vi "Pin Query Context to Channel List.vi"(0 "Pin Query Context":refnum<class "PinQueryContext.lvclass">, 5 "Expanded Pin Information":T1[](array[typedef]), 9 "Site Numbers In":i32[](array[numeric]), 11 "error in":errorcluster) -> (4 "Per-Session Channel List":string[](array[string]), 6 "Pins":tag[](array[tag]), 10 "Site Numbers Out":i32[](array[numeric]), 15 "error out":errorcluster)   [LabVIEW 2020]
uses:
  <vilib>/NI_TestStand_SemiconductorModule/NI_TestStand_Semiconductor_Module.lvlibp/PinMap/PinQueryContext/PinQueryContext.lvclass
  TSM Expanded Pin Information.ctl
  TSM Pin Type Identifier.ctl
  <vilib>/NI_TestStand_SemiconductorModule/NI_TestStand_Semiconductor_Module.lvlibp/PinMap/Advanced/GetPinsInPinGroups.vi
  <vilib>/NI_TestStand_SemiconductorModule/NI_TestStand_Semiconductor_Module.lvlibp
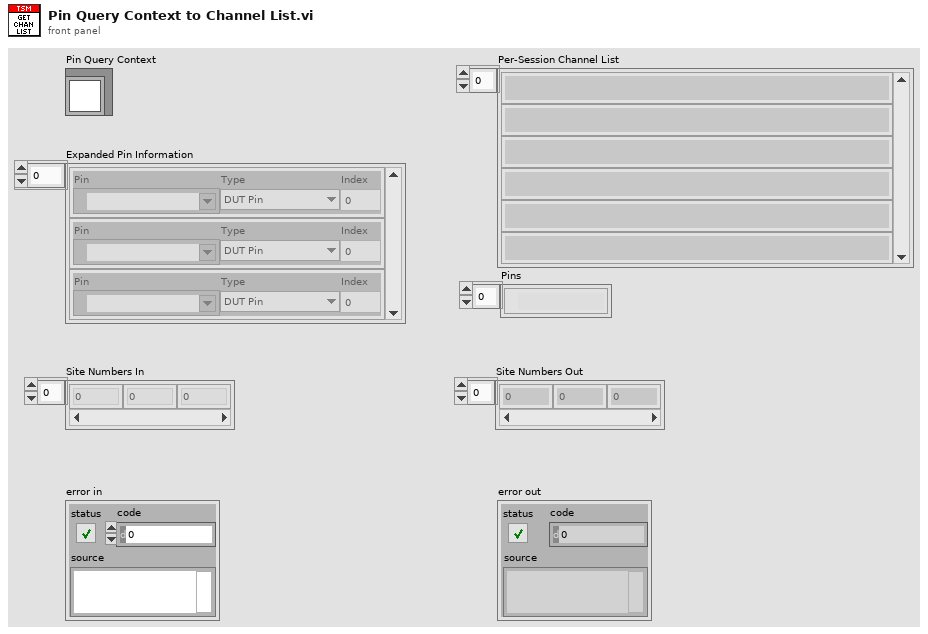
[diagram p1: front panel]
types:
  T1 = typedef "TSM Expanded Pin Information.ctl" = cluster{"Pin":tag, "Type":T2, "Index":i32}
  T2 = typedef "TSM Pin Type Identifier.ctl" = enum8{"DUT Pin", "System Pin", "Pin Group", "Not Determined"}
  T3 = typedef "NI_TestStand_Semiconductor_Module.lvlibp/TSM_Pin.ctl" = tag
  T4 = typedef "NI_TestStand_Semiconductor_Module.lvlibp/SemiconductorModuleContext.ctl" = refnum<k7>
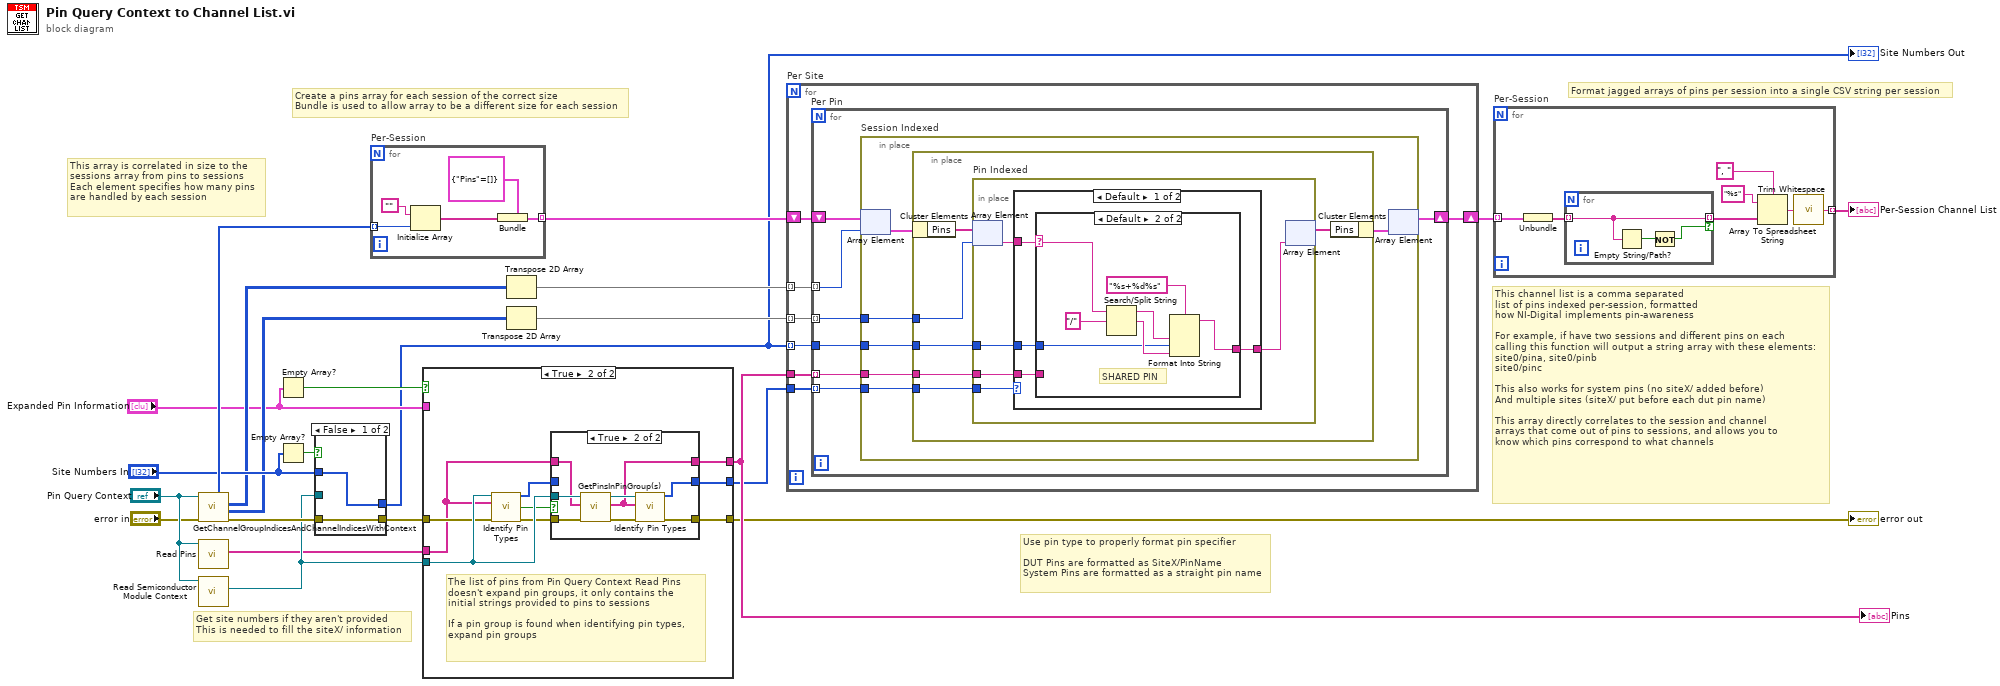
[diagram p0: block diagram]
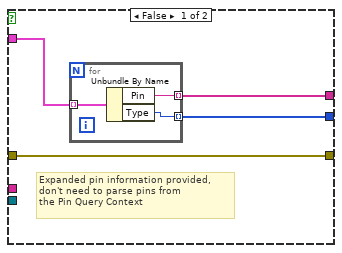
[diagram p2: hidden frame]
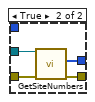
[diagram p4: hidden frame]
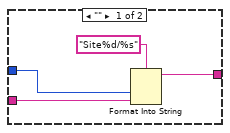
[diagram p5: hidden frame]
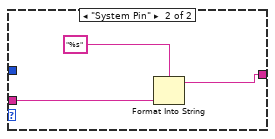
[diagram p6: hidden frame]
diagram:
  # "Use pin type to properly format pin specifier\n\nDUT Pins are formatted as SiteX/PinName\nSystem Pins are formatted as a straight pin name"
  # "Create a pins array for each session of the correct size\nBundle is used to allow array to be a different size for each session"
  # "Format jagged arrays of pins per session into a single CSV string per session"
  # "This array is correlated in size to the \nsessions array from pins to sessions\nEach element specifies how many pins\nare handled by each session"
  # "Get site numbers if they aren't provided\nThis is needed to fill the siteX/ information"
  # "This channel list is a comma separated\nlist of pins indexed per-session, formatted\nhow NI-Digital implements pin-awareness\n\nFor example, if have two sessions and different pins on each\ncalling this function will output a string array with these elements:\nsite0/pina, site0/pinb\nsite0/pinc\n\nThis also works for system pins (no siteX/ added before)\nAnd multiple sites (siteX/ put before each dut pin name)\n\nThis array directly correlates to the session and channel \narrays that come out of pins to sessions, and allows you to\nknow which pins correspond to what channels"
  n1 = call <vilib>:"GetChannelGroupIndicesAndChannelIndicesWithContext.vi"("error in (no error)"="error in", "Publish Token"="Pin Query Context") -> ("error out"=w15:errorcluster, "Channel Indices"=w9:i32[][], "Channel Group Indices"=w10:i32[][], "Number of Pins Per Channel Group"=w17:i32[])  [unwired: 5 in, 1 out]
  n2 = call-dynamic "Read Pins.vi"("Pin Query Context"="Pin Query Context") -> ("Pins"=w7:T3[])  [unwired: 8 in, 2 out]
  n3 = call <vilib>:"Read Semiconductor Module Context.vi"("Pin Query Context"="Pin Query Context") -> ("Semiconductor Module Context"=w11:T4)  [unwired: 8 in, 2 out]
  n4 = Empty Array?(array="Expanded Pin Information") -> (empty?=w3:bool)
  n5 = Empty Array?(array="Site Numbers In") -> (empty?=w13:bool)
  n6 = case shown="False" w13 {
    tunnel: w15 -> [w24 w28]
    tunnel: [w24 w27] -> w8
    tunnel: w11 -> [_ w26]
    tunnel: [w23 w25] -> w1
    tunnel: "Site Numbers In" -> [w23 _]
    frame False {
    }
    frame True {
      n7 = call <vilib>:"GetSiteNumbers.vi"("error in (no error)"=w28, "Semiconductor Module Context"=w26) -> ("error out"=w27:errorcluster, "Site Numbers"=w25:i32[])  [unwired: 6 in, 2 out]
    }
  }
  "Site Numbers Out" <- w1
  n8 = for "Per-Session" {
    tunnel: w17 -> [w32] mode=indexing
    tunnel: [w30] -> w20 mode=indexing
    n9 = Initialize Array("", w32) -> (w31:string[])
    n10 = Bundle(cluster=cluster{"Pins":string[]} {"Pins"=[]}, "Pins"=w31) -> (w30:cluster{"Pins":string[]})
  }
  n11 = case shown="True" w3 {
    tunnel: w11 -> [_ w49]
    tunnel: w8 -> [w34 w48]
    tunnel: w7 -> [_ w44]
    tunnel: [w36 w43] -> w6
    tunnel: [w35 w42] -> w5
    tunnel: [w34 w41] -> w4
    tunnel: "Expanded Pin Information" -> [w37 _]
    frame False {
      # "Expanded pin information provided, \ndon't need to parse pins from \nthe Pin Query Context"
      n12 = for {
        tunnel: w37 -> [w40] mode=indexing
        tunnel: [w39] -> w36 mode=indexing
        tunnel: [w38] -> w35 mode=indexing
        n13 = Unbundle By Name(w40) -> ("Pin"=w39:tag, "Type"=w38:T2)
      }
    }
    frame True {
      # "The list of pins from Pin Query Context Read Pins\ndoesn't expand pin groups, it only contains the \ninitial strings provided to pins to sessions\n\nIf a pin group is found when identifying pin types, \nexpand pin groups"
      n14 = call "Identify Pin Types.vi"("TSM context"=w49, "Pins and/or Pin Groups"=w44, "error in"=w48) -> ("Pin Types"=w45:T2[], "Pin Group Found?"=w47:bool, "error out"=w46:errorcluster)  [unwired: 10 in]
      n15 = case shown="True" w47 {
        tunnel: w49 -> [_ w60]
        tunnel: w46 -> [w50 w54]
        tunnel: w45 -> [w52 _]
        tunnel: w44 -> [w51 w57]
        tunnel: [w52 w56] -> w42
        tunnel: [w51 w55] -> w43
        tunnel: [w50 w53] -> w41
        frame False {
        }
        frame True {
          n16 = call-poly <vilib>:"GetPinsInPinGroup(s).vi"("error in (no error)"=w54, "Pin Groups"=w57, "Semiconductor Module Context"=w60) -> ("error out"=w58:errorcluster, "Pins"=w55:T3[], "Semiconductor Module Context Out"=w59:T4)  [unwired: 6 in]
          n17 = call "Identify Pin Types.vi"("TSM context"=w59, "Pins and/or Pin Groups"=w55, "error in"=w58) -> ("Pin Types"=w56:T2[], "error out"=w53:errorcluster)  [unwired: 10 in, 1 out]
        }
      }
    }
  }
  "error out" <- w4
  "Pins" <- w6
  n18 = Transpose 2D Array(2D array=w10) -> (transposed array=w22:i32[][])
  n19 = Transpose 2D Array(2D array=w9) -> (transposed array=w21:i32[][])
  n20 = for "Per Site" {
    tunnel: w22 -> [w67] mode=indexing
    tunnel: w21 -> [w66] mode=indexing
    shift-right: [w64] -> w19
    shift-left: w20 -> [w65]
    tunnel: w6 -> [w63]
    tunnel: w1 -> [w62] mode=indexing
    tunnel: w5 -> [w61]
    n21 = for "Per Pin" {
      tunnel: w67 -> [w73] mode=indexing
      tunnel: w66 -> [w72] mode=indexing
      shift-right: [w71] -> w64
      shift-left: w65 -> [w74]
      tunnel: w63 -> [w70] mode=indexing
      tunnel: w62 -> [w69]
      tunnel: w61 -> [w68] mode=indexing
      n22 = in-place "Session Indexed" {
        in-place-border: w72 -> [w79]
        in-place-border: w70 -> [w78]
        in-place-border: w69 -> [w76]
        in-place-border: w68 -> [w75]
        n23 = in-place-array #1(w74, w73) -> (w80:cluster{"Pins":string[]})
        n24 = in-place {
          in-place-border: w79 -> [w85]
          in-place-border: w78 -> [w84]
          in-place-border: w76 -> [w82]
          in-place-border: w75 -> [w81]
          n25 = in-place-cluster #2(w80) -> ("Pins"=w86:string[])
          n26 = in-place "Pin Indexed" {
            in-place-border: w84 -> [w91]
            in-place-border: w82 -> [w90]
            in-place-border: w81 -> [w88]
            n27 = in-place-array #3(w86, w85) -> (w87:string)
            n28 = case shown="Default" w88 {
              tunnel: w91 -> [w95 w109]
              tunnel: w90 -> [w94 _]
              tunnel: [w93 w108] -> w89
              tunnel: w87 -> [w92 _]
              frame Default {
                n29 = case shown="Default" w92 {
                  selector: w92 -> [_ w106]
                  tunnel: w95 -> [w99 _]
                  tunnel: w94 -> [w98 w102]
                  tunnel: [w97 w101] -> w93
                  frame "" {
                    n30 = Format Into String(format string="Site%d/%s", w98, w99) -> (resulting string=w97:string)  [unwired: 2 in, 1 out]
                  }
                  frame Default {
                    # "SHARED PIN"
                    n31 = Search/Split String(string=w106, search string/char (-)="/") -> (substring before match=w104:string, match + rest of string=w103:string)  [unwired: 1 in, 1 out]
                    n32 = Format Into String(format string="%s+%d%s", w104, w102, w103) -> (resulting string=w101:string)  [unwired: 2 in, 1 out]
                  }
                }
              }
              frame "System Pin" {
                n33 = Format Into String(format string="%s", w109) -> (resulting string=w108:string)  [unwired: 2 in, 1 out]
              }
            }
            n34 = in-place-array #3(w89) -> (w83:string[])  [unwired: 1 out]
          }
          n35 = in-place-cluster #2("Pins"=w83) -> (w77:cluster{"Pins":string[]})
        }
        n36 = in-place-array #1(w77) -> (w71:cluster{"Pins":string[]}[])  [unwired: 1 out]
      }
    }
  }
  n37 = for "Per-Session" {
    tunnel: w19 -> [w116] mode=indexing
    tunnel: [w112] -> w18 mode=indexing
    n38 = Unbundle(w116) -> ("Pins"=w111:string[])
    n39 = for {
      tunnel: w111 -> [w119] mode=indexing
      tunnel: [w119] -> w110 mode=indexing if=w117
      n40 = Empty String/Path?(string/path=w119) -> (empty?=w118:bool)
      n41 = Not(x=w118) -> (.not. x?=w117:bool)
    }
    n42 = Array To Spreadsheet String(delimiter (Tab)=", ", array=w110, 3:"%s" ("format string")) -> (spreadsheet string=w113:string)
    n43 = call <vilib>:"Trim Whitespace.vi"("string"=w113) -> ("trimmed string"=w112:string)  [unwired: 1 in]
  }
  "Per-Session Channel List" <- w18
